vi "InitDevice.vi"(7 "ID(Hex 高位有效)":string="002", 8 "错误输入（无错误）":errorcluster, 9 "InitConfig":T2={"AccCode"=0, "AccMask"=4294967295, "Reserved"=0, "Filter"=0, "kCanBaud"=12, "Timing0"=10, "Timing1"=0, "Mode"=0, "CanRx_IER"=1} {"CanRx_IER" items=["0", "1"]; "kCanBaud" items=["250k bps"=10, "10k bps"=2, "5k bps"=1, "50k bps"=5, "40k bps"=4, "20k bps"=3, "80k bps"=6, "100k bps"=7, "125k bps"=8, "200k bps"=9, "400k bps"=11, "500k bps"=12, "666k bps"=13, "800k bps"=14, "1000k bps"=15]; "Mode" items=["Normal", "Self TX-RX"]; "Filter" items=["Single Filter", "Dual Filter"]; "AccCode" format="%08x"; "AccMask" format="%08x"; "Timing0" format="%02x"; "Timing1" format="%02x"}, 10 "CanChannel":u32, 11 "DeviceType":T1=3 items=["PCI-CAN200"=7, "USB-CAN"=2, "USB-CAN200"=3]) -> (0 "错误输出":errorcluster, 2 "Result":bool, 3 "DeviceTypeOut":u16(ring)=7 items=["PCI-CAN200"=7])   [LabVIEW 2013]
uses:
  InitConfig.ctl
  DevType.ctl
  VCI_CAN.dll
panel:
  out "屏蔽码":u32 format="%.0x"
  out "验收码":u32 format="%.0x"
  in  "滤波":bool=TRUE
  out "输出簇":T2={"AccCode"=0, "AccMask"=4294967295, "Reserved"=0, "Filter"=0, "kCanBaud"=10, "Timing0"=0, "Timing1"=0, "Mode"=0, "CanRx_IER"=0} {"CanRx_IER" items=["0", "1"]; "kCanBaud" items=["250k bps"=10, "10k bps"=2, "5k bps"=1, "50k bps"=5, "40k bps"=4, "20k bps"=3, "80k bps"=6, "100k bps"=7, "125k bps"=8, "200k bps"=9, "400k bps"=11, "500k bps"=12, "666k bps"=13, "800k bps"=14, "1000k bps"=15]; "Mode" items=["Normal", "Self TX-RX"]; "Filter" items=["Single Filter", "Dual Filter"]; "AccCode" format="%08x"; "AccMask" format="%08x"; "Timing0" format="%02x"; "Timing1" format="%02x"}
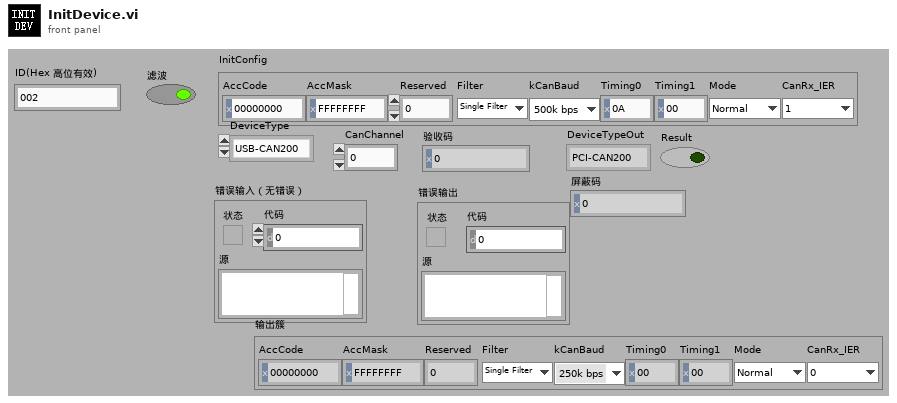
[diagram p1: front panel]
types:
  T1 = typedef "DevType.ctl" = u16
  T2 = typedef "InitConfig.ctl" = cluster{"AccCode":u32, "AccMask":u32, "Reserved":u32, "Filter":u8, "kCanBaud":u8, "Timing0":u8, "Timing1":u8, "Mode":u8, "CanRx_IER":u8}
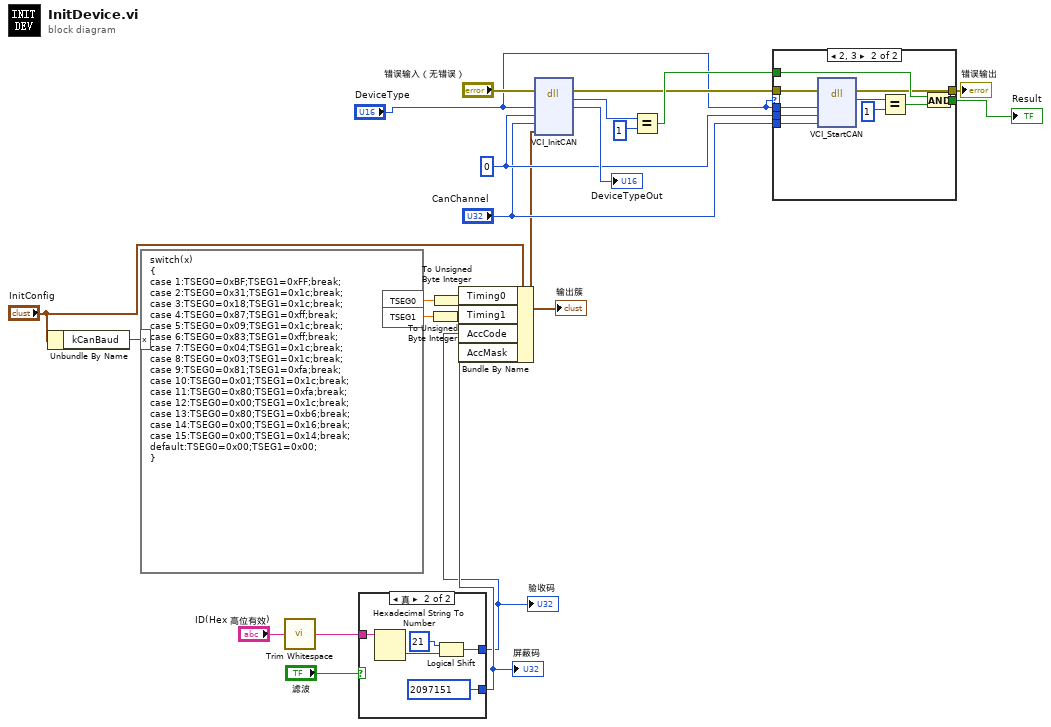
[diagram p0: block diagram]
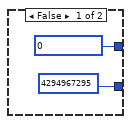
[diagram p2: hidden frame]
diagram:
  w13 = 0
  n1 = Unbundle By Name("InitConfig") -> ("kCanBaud"=w19:u8)
  n2 = formula code="switch(x)\n{ \ncase 1:TSEG0=0xBF;TSEG1=0xFF;break;\ncase 2:TSEG0=0x31;TSEG1=0x1c;break;\ncase 3:TSEG0=0x18;TSEG1=0x1c;break;\ncase 4:TSEG0=0x87;TSEG1=0xff;break;\ncase 5:TSEG0=0x09;TSEG1=0x1c;break;\ncase 6:TSEG0=0x83;TSEG1=0xff;break;\ncase 7:TSEG0=0x04;TSEG1=0x1c;break;\ncase 8:TSEG0=0x03;TSEG1=0x1c;break;\ncase 9:TSEG0=0x81;TSEG1=0xfa;break;\ncase 10:TSEG0=0x01;TSEG1=0x1c;break;\ncase 11:TSEG0=0x80;TSEG1=0xfa;break;\ncase 12:TSEG0=0x00;TSEG1=0x1c;break;\ncase 13:TSEG0=0x80;TSEG1=0xb6;break;\ncase 14:TSEG0=0x00;TSEG1=0x16;break;\ncase 15:TSEG0=0x00;TSEG1=0x14;break;\ndefault:TSEG0=0x00;TSEG1=0x00;\n}"("x"=w19) -> ("TSEG0"=w17:dbl, "TSEG1"=w18:dbl)
  n3 = call <vilib>:"Trim Whitespace.vi"("string"="ID(Hex 高位有效)") -> ("trimmed string"=w4:string)  [unwired: 1 in]
  n4 = case shown="真" "滤波" {
    tunnel: w4 -> [_ w29]
    tunnel: [u32 0 ("验收码") w26] -> w1
    tunnel: [u32 4294967295 ("屏蔽码") u32 2097151 ("屏蔽码")] -> w2
    frame False {
    }
    frame True {
      n5 = Hexadecimal String To Number(string=w29) -> (number=w27:u32)  [unwired: 2 in, 1 out]
      n6 = Logical Shift(y=i8 21, x=w27) -> (x << y=w26:u32)
    }
  }
  "验收码" <- w1
  "屏蔽码" <- w2
  n7 = To Unsigned Byte Integer(number=w18) -> (unsigned 8bit integer=w15:u8)
  n8 = To Unsigned Byte Integer(number=w17) -> (unsigned 8bit integer=w16:u8)
  n9 = Bundle By Name(cluster="InitConfig", "Timing0"=w16, "Timing1"=w15, "AccCode"=w1, "AccMask"=w2) -> (w6:T2)
  "输出簇" <- w6
  n10 = dll-call lib="PTH1abs CUsers\nAdministratorDesktop360æºç åå¤360å¨æ¯ä¸»æºæåæµè¯V816InstrumentDriversUSB-CANVCI_CAN.dll" fn="VCI_InitCAN"(error in="错误输入（无错误）", "DevType"="DeviceType", "DevIndex"=w13, "CanIndex"="CanChannel", "pInitConfig"=w6) -> (error out=w9:errorcluster, "返回类型"=w22:u32, "DevType"=→"DeviceTypeOut":u32)  [unwired: 5 in, 1 out]
  n11 = Equal?(x=w22, y=u32 1) -> (x = y?=w11:bool)
  n12 = case shown="2, 3" "DeviceType" {
    tunnel: "DeviceType" -> [_ w42]
    tunnel: w13 -> [_ w41]
    tunnel: "CanChannel" -> [_ w40]
    tunnel: w11 -> [w31 w37]
    tunnel: [w31 w35] -> w10
    tunnel: w9 -> [w32 w34]
    tunnel: [w32 w33] -> w8
    frame 0, Default {
    }
    frame 2, 3 {
      n13 = dll-call lib="PTH1abs CUsers\nAdministratorDesktop360æºç åå¤360å¨æ¯ä¸»æºæåæµè¯V816InstrumentDriversUSB-CANVCI_CAN.dll" fn="VCI_StartCAN"(error in=w34, "DeviceType"=w42, "DeciceInd"=w41, "CANInd"=w40) -> (error out=w33:errorcluster, "返回类型"=w39:u32)  [unwired: 5 in, 1 out]
      n14 = Equal?(x=w39, y=u32 1) -> (x = y?=w36:bool)
      n15 = And(x=w37, y=w36) -> (x .and. y?=w35:bool)
    }
  }
  "错误输出" <- w8
  "Result" <- w10
